vi "GetConnectStatus.vi"(8 "error in (no error)":errorcluster, 11 "SharedVariableWrapper in":refnum<class "SharedVariableWrapper.lvclass">) -> (0 "error out":errorcluster, 1 "map":map{string, T1}(c390), 2 "Connected?":bool)   [LabVIEW 2019, in "SharedVariableWrapper.lvclass"]
uses:
  SharedVariableWrapper.lvclass
  shared variable info.ctl
  SharedVariableWrapper.lvclass/SharedVariableWrapper.ctl
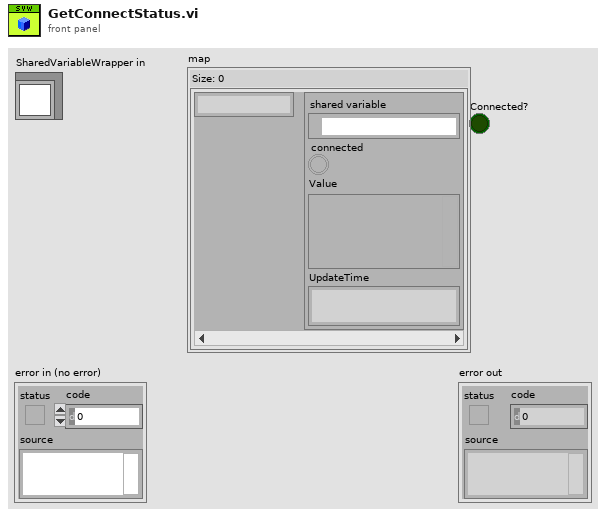
[diagram p1: front panel]
types:
  T1 = typedef "SharedVariableWrapper.lvclass/shared variable info.ctl" = cluster{"shared variable":refnum<k21>, "connected":bool, "Value":variant, "UpdateTime":timestamp}
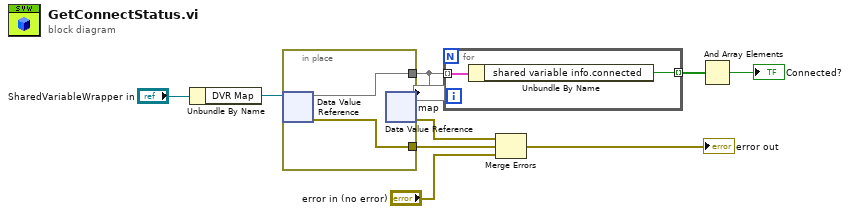
[diagram p0: block diagram]
diagram:
  n1 = Unbundle By Name("SharedVariableWrapper in") -> ("DVR Map"=w7:refnum<data-value>)
  n2 = in-place {
    in-place-border: [w11] -> w4
    in-place-border: [w10] -> w6
    n3 = in-place-dvr #1(w7) -> (w10:map{string, T1}, w11:errorcluster)
    n4 = in-place-dvr #1() -> (w5:errorcluster)  [unwired: 1 in, 1 out]
  }
  "map" <- w6
  n5 = for {
    tunnel: w6 -> [w13] mode=indexing
    tunnel: [w12] -> w2 mode=indexing
    n6 = Unbundle By Name(w13) -> ("shared variable info.connected"=w12:bool)
  }
  n7 = Merge Errors(w5, w4, "error in (no error)") -> (→"error out":errorcluster)
  n8 = And Array Elements(Boolean array=w2) -> (logical AND=→"Connected?":bool)
